vi "Fibonacci_series.vi"() -> ()   [LabVIEW 2019]
panel:
  out "Numeric":u64
  out "Array form":u64[](array[numeric])
  in  "stop":bool
  out "Fibonacci series":u64
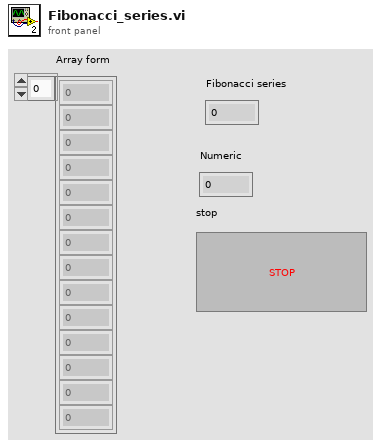
[diagram p1: front panel]
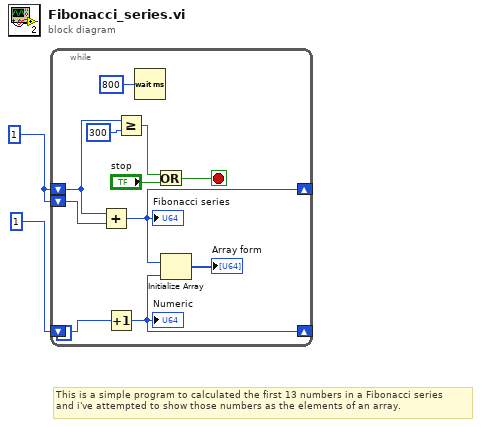
[diagram p0: block diagram]
diagram:
  w2 = u64 1
  # "This is a simple program to calculated the first 13 numbers in a Fibonacci series\nand i've attempted to show those numbers as the elements of an array."
  n1 = while {
    shift-right: [w3] -> _
    shift-left: w2 -> [w11]
    shift-left: w2 -> [w13]
    shift-right: [w5] -> _
    shift-left: u64 1 -> [w6]
    stop <- w8 stop-if-true
    n2 = Add(x=w11, y=w13) -> (x+y=w3:u64)
    "Fibonacci series" <- w3
    n3 = Increment(x=w6) -> (x+1=w5:u64)
    "Numeric" <- w5
    n4 = Greater Or Equal?(x=w11, y=u64 300) -> (x >= y?=w9:bool)
    n5 = Wait (ms)(milliseconds to wait=u32 800) -> ()  [unwired: 1 out]
    n6 = Or(x=w9, y="stop") -> (x .or. y?=w8:bool)
    n7 = Initialize Array(w3, w5) -> (→"Array form":u64[])
  }
